vi "test register module.vi"() -> ()   [LabVIEW 2017]
uses:
  user.lib/_NEVSTOP/Communicable State Machine(CSM)/AdvanceAPI/CSM - Broadcast Message Type.ctl
  user.lib/_NEVSTOP/Communicable State Machine(CSM)/_Support/ChangeFlag/FlagInstance-CSMQ FGV.vi
  user.lib/_NEVSTOP/Communicable State Machine(CSM)/_Support/ChangeFlag/FlagInstance-Broadcast Cache.vi
  user.lib/_NEVSTOP/Communicable State Machine(CSM)/_Support/ChangeFlag/ChangeFlag-Read.vi
  user.lib/_NEVSTOP/Communicable State Machine(CSM)/_Support/ChangeFlag/ChangeFlagDB.vi
  user.lib/_NEVSTOP/Communicable State Machine(CSM)/_Shared/Trim Single-line Text.vi
  user.lib/_NEVSTOP/Communicable State Machine(CSM)/_Support/BroadcastRegistry/HelperVI/Broadcast Item Key.vi
  user.lib/_NEVSTOP/Communicable State Machine(CSM)/_Support/FGV-BroadcastRegistry/FGV-BroadcastRegistry(lvlibp).vi
  user.lib/_NEVSTOP/Communicable State Machine(CSM)/Communicable State Machine.lvlib
panel:
  out "Array":T2(array[cluster])
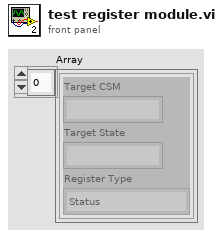
[diagram p1: front panel]
types:
  T1 = typedef "Communicable State Machine.lvlib/CSM - Broadcast Message Type.ctl" = enum16{"<Null>", "Status", "Interrupt"}
  T2 = cluster{"Target CSM":string, "Target State":string, "Register Type":T1}[]
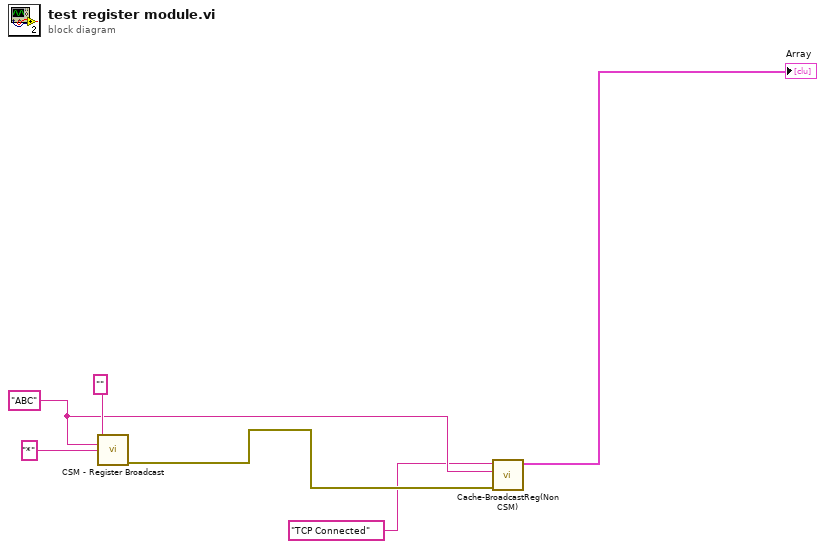
[diagram p0: block diagram]
diagram:
  w2 = "ABC" ("Source CSM Name (* as Default)")
  n1 = call "CSM - Register Broadcast.vi"("CSM Name(Empty for Broadcast Event)"="" ("CSM Name"), "Source CSM Name (* as Default)"=w2, "Trigger"="*") -> ("error out"=w5:errorcluster)  [unwired: 11 in, 1 out]
  n2 = call "Cache-BroadcastReg(NonCSM).vi"("error in (no error)"=w5, "CSM Name"=w2, "Broadcast State"="TCP Connected" ("CSM Name")) -> ("Array"=→"Array":T2)  [unwired: 7 in, 1 out]
